vi "Test_URI Parsing.vi"(8 "error in (no error)":errorcluster) -> (0 "error out":errorcluster)   [LabVIEW 2013]
uses:
  <vilib>/addons/_JKI Toolkits/Caraya/classes/Assert/Assert Equal Value_Variant.vi
  <vilib>/addons/_JKI Toolkits/Caraya/classes/Assert/Assert True.vi
  <vilib>/Utility/error.llb/Trim Whitespace.vi
  source/utilities/Extract URI Components.vi
  source/openURI.lvlib
  <vilib>/addons/_JKI Toolkits/Caraya/classes/Test/Test.lvclass
  <vilib>/addons/_JKI Toolkits/Caraya/classes/Assert/Assert.lvclass
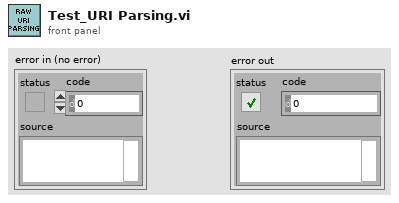
[diagram p1: front panel]
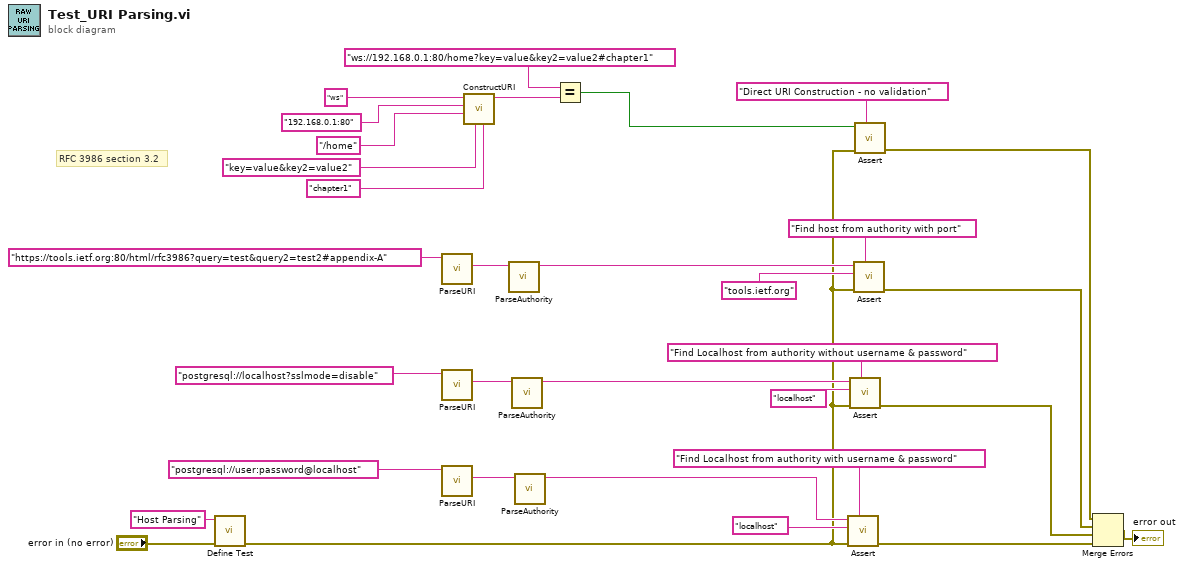
[diagram p0: block diagram]
diagram:
  # "RFC 3986 section 3.2"
  n1 = call <vilib>:"Define Test.vi"("error in (no error)"="error in (no error)", "Label (VI Title)"="Host Parsing") -> ("error out"=w3:errorcluster)  [unwired: 9 in]
  n2 = call "ParseURI.vi"("URI"="https://tools.ietf.org:80/html/rfc3986?query=test&query2=test2#appendix-A") -> ("authority"=w15:string)  [unwired: 5 in, 5 out]
  n3 = call "ParseURI.vi"("URI"="postgresql://localhost?sslmode=disable") -> ("authority"=w17:string)  [unwired: 5 in, 5 out]
  n4 = call "ParseURI.vi"("URI"="postgresql://user:password@localhost") -> ("authority"=w19:string)  [unwired: 5 in, 5 out]
  n5 = call "ConstructURI.vi"("fragment"="chapter1" ("URI"), "query"="key=value&key2=value2" ("URI"), "path component"="/home" ("URI"), "authority"="192.168.0.1:80" ("URI"), "scheme"="ws") -> ("URI"=w6:string)  [unwired: 5 in, 1 out]
  n6 = call "ParseAuthority.vi"("authority"=w15) -> ("host"=w14:string)  [unwired: 7 in, 3 out]
  n7 = call "ParseAuthority.vi"("authority"=w17) -> ("host"=w16:string)  [unwired: 7 in, 3 out]
  n8 = call "ParseAuthority.vi"("authority"=w19) -> ("host"=w18:string)  [unwired: 7 in, 3 out]
  n9 = Equal?(x="ws://192.168.0.1:80/home?key=value&key2=value2#chapter1" ("URI"), y=w6) -> (x = y?=w4:bool)
  n10 = call-poly <vilib>:"Assert.vi"("Label"="Find Localhost from authority with username & password" ("URI"), "error in (no error)"=w3, "Y"="localhost" ("URI"), "X"=w18) -> ("error out"=w24:errorcluster)  [unwired: 7 in]
  n11 = call-poly <vilib>:"Assert.vi"("Label"="Find Localhost from authority without username & password" ("URI"), "error in (no error)"=w3, "Y"="localhost" ("URI"), "X"=w16) -> ("error out"=w23:errorcluster)  [unwired: 7 in]
  n12 = call-poly <vilib>:"Assert.vi"("Label"="Find host from authority with port" ("URI"), "error in (no error)"=w3, "Y"="tools.ietf.org" ("URI"), "X"=w14) -> ("error out"=w20:errorcluster)  [unwired: 7 in]
  n13 = call-poly <vilib>:"Assert.vi"("Label"="Direct URI Construction - no validation" ("URI"), "error in (no error)"=w3, "True?"=w4) -> ("error out"=w2:errorcluster)  [unwired: 8 in]
  n14 = Merge Errors(w2, w20, w23, w24) -> (→"error out":errorcluster)
